vi "generate vi error list.vi"(8 "error in (no error)":errorcluster, 10 "get vi error list Argument":T2, 11 "Data Cluster in":T1) -> (0 "error out":errorcluster, 2 "Error Description":string, 3 "Data Cluster out":T1)   [LabVIEW 2025, in "Scripting Server.lvlib"]
uses:
  Scripting Server.lvlib
  Module Data--cluster.ctl
  get vi error list Argument--cluster.ctl
  get vi error list (Reply Payload)--cluster.ctl
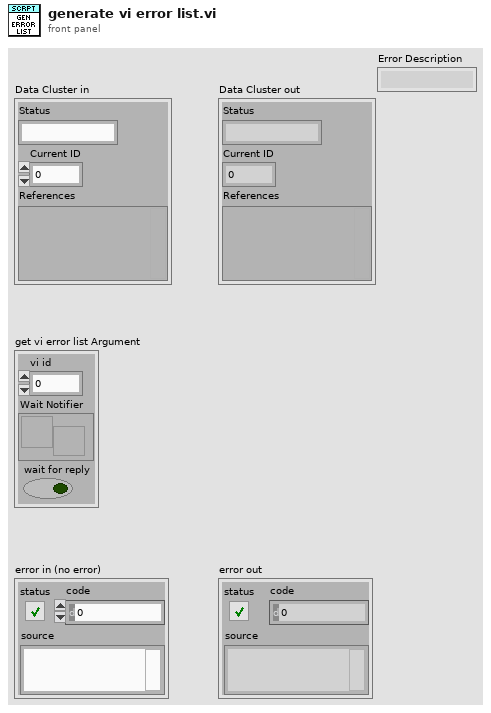
[diagram p1: front panel]
types:
  T1 = typedef "Scripting Server.lvlib/Module Data--cluster.ctl" = cluster{"Status":string, "Current ID":i32, "References":variant}
  T2 = typedef "Scripting Server.lvlib/get vi error list Argument--cluster.ctl" = cluster{"vi id":i32, "Wait Notifier":refnum<notifier>, "wait for reply":bool}
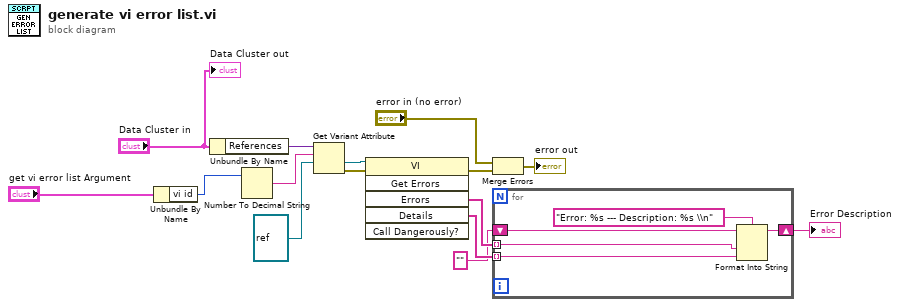
[diagram p0: block diagram]
diagram:
  n1 = Unbundle By Name("get vi error list Argument") -> ("vi id"=w10:i32)
  n2 = Unbundle By Name("Data Cluster in") -> ("References"=w11:variant)
  n3 = Number To Decimal String(number=w10) -> (decimal integer string=w9:string)  [unwired: 1 in]
  n4 = Get Variant Attribute(Variant=w11, name=w9, default value (empty Variant)=refnum<vi> refnum ("vi refnum")) -> (value=w1:refnum<vi>, error out=w7:errorcluster)  [unwired: 1 in, 2 out]
  n5 = invoke class="VI" method="Get Errors"(reference=w1, error in=w7) -> (error out=w4:errorcluster, "Errors"=w6:string[], "Details"=w5:string[])  [unwired: 4 in, 3 out]
  n6 = Merge Errors("error in (no error)", w4) -> (→"error out":errorcluster)
  n7 = for {
    tunnel: w6 -> [w17] mode=indexing
    tunnel: w5 -> [w16] mode=indexing
    shift-right: [w20] -> w2
    shift-left: "" -> [w19]
    n8 = Format Into String(format string="Error: %s --- Description: %s \\n", initial string=w19, w17, w16) -> (resulting string=w20:string)  [unwired: 1 in, 1 out]
  }
  "Error Description" <- w2
  "Data Cluster out" <- "Data Cluster in"
